vi "User Update for Spartan 5.0.vi"(8 "error in (no error)":errorcluster, 10 "Old User Record":T1) -> (0 "error out":errorcluster, 2 "New User Record":T1)   [LabVIEW 2011]
uses:
  User Record.ctl
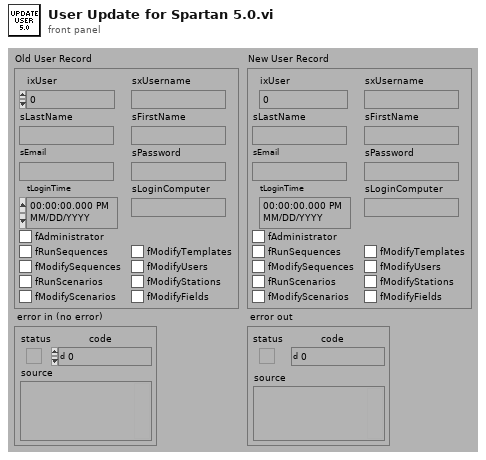
[diagram p1: front panel]
types:
  T1 = typedef "User Record.ctl" = cluster{"ixUser":i32, "sxUsername":string, "sLastName":string, "sFirstName":string, "sEmail":string, "sPassword":string, "tLoginTime":timestamp, "sLoginComputer":string, "fAdministrator":bool, "fRunSequences":bool, "fModifySequences":bool, "fRunScenarios":bool, "fModifyScenarios":bool, "fModifyTemplates":bool, "fModifyUsers":bool, "fModifyStations":bool, "fModifyFields":bool}
  T2 = typedef "User Permissions.ctl" = cluster{"Run Tests":bool, "Edit Sequences":bool, "View Results":bool, "System":bool, "Edit Users":bool, "Edit Stations":bool, "Edit Instruments":bool, "Edit Database":bool, "Sample Testing":bool}
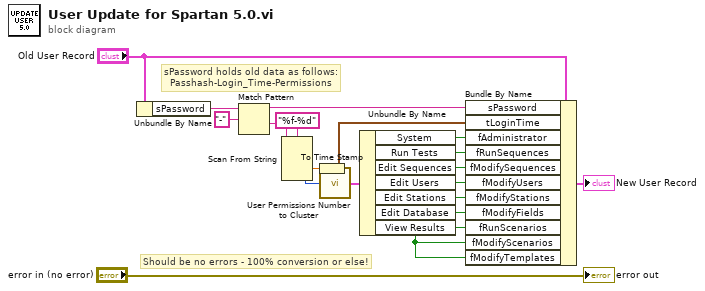
[diagram p0: block diagram]
diagram:
  # "sPassword holds old data as follows:\n  Passhash-Login_Time-Permissions"
  # "Should be no errors - 100% conversion or else!"
  n1 = Unbundle By Name("Old User Record") -> ("sPassword"=w14:string)
  n2 = Match Pattern(string=w14, regular expression="-") -> (before substring=w12:string, after substring=w15:string)  [unwired: 3 out]
  n3 = Scan From String(format string="%f-%d", input string=w15) -> (output 1=w11:dbl, output 2=w9:i32)  [unwired: 2 in, 5 out]
  n4 = To Time Stamp(1:w11) -> (0:w10:timestamp)
  n5 = call "User Permissions Number to Cluster.vi"("User Permissions"=w9) -> ("User Permisions"=w8:T2)
  n6 = Unbundle By Name(w8) -> ("System"=w5:bool, "Run Tests"=w7:bool, "Edit Sequences"=w6:bool, "Edit Users"=w4:bool, "Edit Stations"=w3:bool, "Edit Database"=w2:bool, "View Results"=w1:bool)
  n7 = Bundle By Name(cluster="Old User Record", "sPassword"=w12, "tLoginTime"=w10, "fAdministrator"=w5, "fRunSequences"=w7, "fModifySequences"=w6, "fModifyUsers"=w4, "fModifyStations"=w3, "fModifyFields"=w2, "fRunScenarios"=w1, "fModifyScenarios"=w1, "fModifyTemplates"=w1) -> (→"New User Record":T1)
  "error out" <- "error in (no error)"
